vi "Initialize.vi"(7 "Serial Configuration":T1={"Baud Rate"=9600, "Parity"=0, "Data Bits"=8, "Stop Bits"=10, "Flow Control"=0} {"Flow Control" items=["None", "XON/XOFF", "RTS/CTS", "XON/XOFF & RTS/CTS", "DTR/DSR", "XON/XOFF & DTR/DSR"]; "Stop Bits" items=["1.0"=10, "1.5"=15, "2.0"=20]; "Data Bits" items=["7"=7, "8"=8]; "Parity" items=["None", "Odd", "Even", "Mark", "Space"]; "Baud Rate" items=["300"=300, "600"=600, "1200"=1200, "2400"=2400, "4800"=4800, "9600"=9600, "19200"=19200]}, 8 "error in (no error)":errorcluster, 9 "Reset (True)":bool=TRUE, 10 "ID Query (True)":bool=TRUE, 11 "VISA resource name":refnum<visa-resource-name>) -> (0 "error out":errorcluster, 3 "VISA resource name out":refnum<visa-resource-name>)   [LabVIEW 2024, in "Keithley 648X Series.lvlib"]
doc: "Establishes communication with the instrument and optionally performs an instrument identification query and/or an instrument reset. It also places the instrument in a default state needed for other instrument driver operations. Therefore, call this VI before calling other instrument driver VIs for this instrument. Generally, you need to call the <b>Initialize</b> VI only once at the beginning of an application."
uses:
  <instrlib>/Keithley 648X Series/Keithley 648X Series.lvlib
panel:
  # "(c) 2017 National Instruments.  ALL RIGHTS RESERVED."
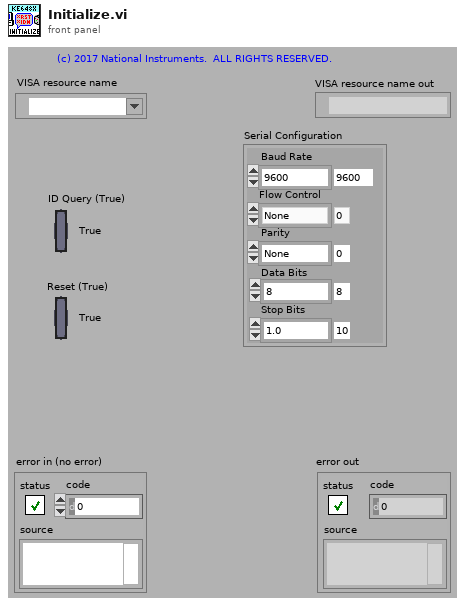
[diagram p1: front panel]
types:
  T1 = cluster{"Baud Rate":u32, "Parity":u16, "Data Bits":u16, "Stop Bits":u16, "Flow Control":u16}
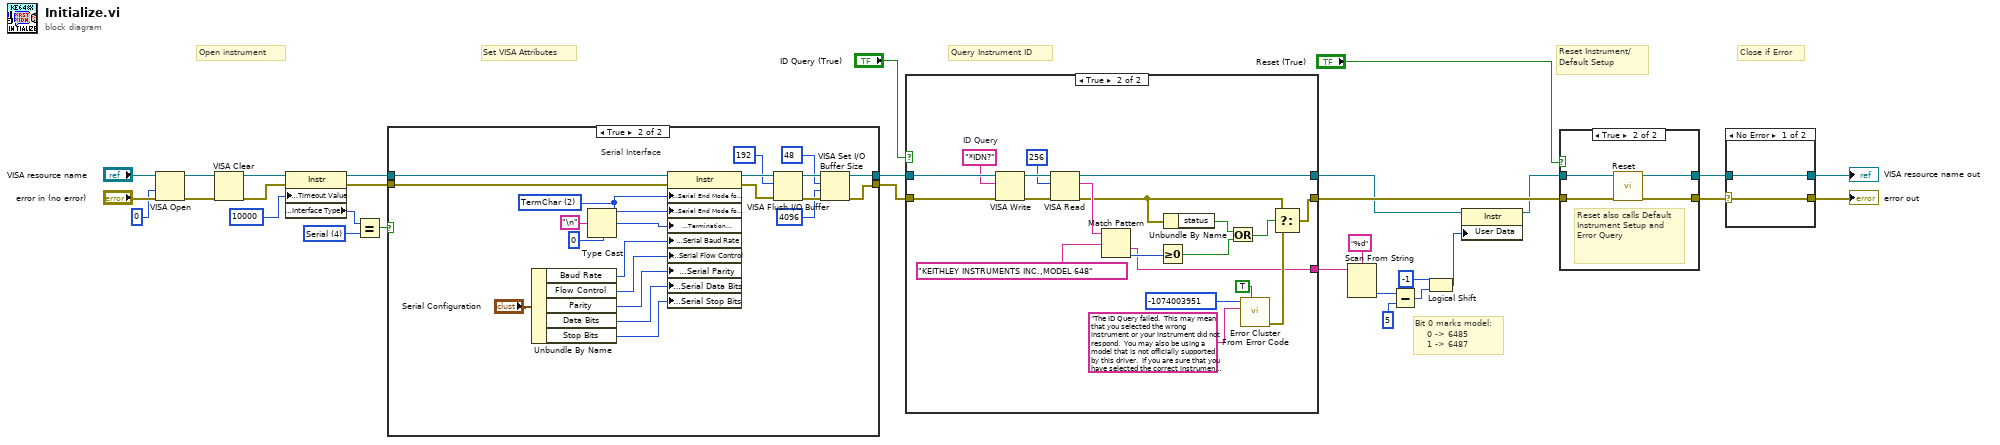
[diagram p0: block diagram]
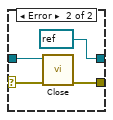
[diagram p3: hidden frame]
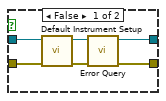
[diagram p4: hidden frame]
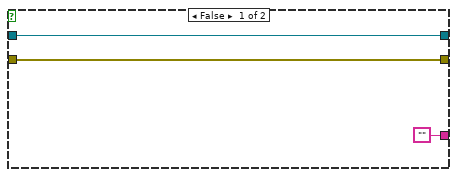
[diagram p5: hidden frame]
diagram:
  w19 = u16 4 items=["GPIB"=1, "VXI"=2, "GPIB-VXI"=3, "Serial"=4, "PXI"=5, "TCPIP"=6, "USB"=7] ("Interface Information:Interface Type")
  # "Bit 0 marks model:\n    0 -> 6485\n    1 -> 6487"
  # "Set VISA Attributes"
  # "Close if Error"
  # "Query Instrument ID"
  # "Reset Instrument/\nDefault Setup"
  # "Open instrument"
  n1 = VISA Open(access mode=u32 0, error in (no error)="error in (no error)", VISA resource name="VISA resource name") -> (VISA resource name=w17:refnum<visa-resource-name>, error out=w16:errorcluster)  [unwired: 2 in]
  n2 = VISA Clear(VISA resource name=w17, error in (no error)=w16) -> (VISA resource name out=w15:refnum<visa-resource-name>, error out=w14:errorcluster)
  n3 = property class="Instr"(reference=w15, error in=w14, "General Settings:Timeout Value"=u32 10000) -> (reference out=w22:refnum<visa-resource-name>, error out=w21:errorcluster, "Interface Information:Interface Type"=w26:u16)
  n4 = Equal?(x=w26, y=w19) -> (x = y?=w20:bool)
  n5 = case shown="True" w20 {
    tunnel: [w32 w51] -> w24
    tunnel: [w33 w48] -> w23
    tunnel: w22 -> [w32 w53]
    tunnel: w21 -> [w33 w54]
    frame False {
      # "GPIB Interface"
    }
    frame True {
      w41 = u16 2 items=["None", "LastBit", "TermChar"] ("Serial Settings:Serial End Mode for Reads")
      # "Serial Interface"
      n6 = Unbundle By Name("Serial Configuration") -> ("Baud Rate"=w39:u32, "Flow Control"=w35:u16, "Parity"=w37:u16, "Data Bits"=w38:u16, "Stop Bits"=w34:u16)
      n7 = Type Cast(type=u8 0, x="\n" ("Line Feed Constant")) -> (*(type *) &x=w40:u8)
      n8 = property class="Instr"(reference=w53, error in=w54, "Serial Settings:Serial End Mode for Reads"=w41, "Serial Settings:Serial End Mode for Writes"=w41, "Message Based Settings:Termination Character"=w40, "Serial Settings:Serial Baud Rate"=w39, "Serial Settings:Serial Flow Control"=w35, "Serial Settings:Serial Parity"=w37, "Serial Settings:Serial Data Bits"=w38, "Serial Settings:Serial Stop Bits"=w34) -> (reference out=w47:refnum<visa-resource-name>, error out=w50:errorcluster)
      n9 = VISA Flush I/O Buffer(VISA resource name=w47, mask (16)=u16 192, error in (no error)=w50) -> (VISA resource name out=w52:refnum<visa-resource-name>, error out=w49:errorcluster)
      n10 = VISA Set I/O Buffer Size(VISA resource name=w52, mask (16)=u16 48, size (4096)=u32 4096 ("size (0)"), error in (no error)=w49) -> (VISA resource name out=w51:refnum<visa-resource-name>, error out=w48:errorcluster)
    }
  }
  n11 = case shown="True" "ID Query (True)" {
    tunnel: [w56 w77] -> w31
    tunnel: [w57 w74] -> w7
    tunnel: w24 -> [w57 w75]
    tunnel: w23 -> [w56 w76]
    tunnel: ["" w58] -> w9
    frame False {
    }
    frame True {
      w68 = "*IDN?"  # ID Query
      n12 = VISA Write(VISA resource name=w75, write buffer=w68, error in (no error)=w76) -> (VISA resource name out=w72:refnum<visa-resource-name>, error out=w71:errorcluster)  [unwired: 1 out]
      n13 = VISA Read(VISA resource name=w72, byte count=u32 256, error in (no error)=w71) -> (VISA resource name out=w74:refnum<visa-resource-name>, read buffer=w73:string, error out=w63:errorcluster)  [unwired: 1 out]
      n14 = Match Pattern(string=w73, regular expression="KEITHLEY INSTRUMENTS INC.,MODEL 648") -> (after substring=w58:string, offset past match=w64:i32)  [unwired: 1 in, 2 out]
      n15 = Greater Or Equal To 0?(x=w64) -> (x >= 0?=w61:bool)
      n16 = Unbundle By Name(w63) -> ("status"=w62:bool)
      n17 = Or(x=w62, y=w61) -> (x .or. y?=w60:bool)
      n18 = call <vilib>:"Error Cluster From Error Code.vi"("show call chain? (False)"=TRUE, "error message (\"\")"="The ID Query failed.  This may mean that you selected the wrong instrument or your instrument did not respond.  You may also be using a model that is not officially supported by this driver.  If you are sure that you have selected the correct instrument and it is responding, try disabling the ID Query." ("Source (VI Name)"), "error code (0)"=-1074003951 ("Code")) -> ("error out"=w67:errorcluster)  [unwired: 6 in]
      n19 = Select(t=w63, s=w60, f=w67) -> (s? t:f=w77:errorcluster)
    }
  }
  n20 = Scan From String(format string="%d", input string=w9) -> (output 1=w6:i32)  [unwired: 3 in, 3 out]
  n21 = Subtract(x=w6, y=5) -> (x-y=w3:i32)
  n22 = Logical Shift(y=i16 -1, x=w3) -> (x << y=w4:i32)
  n23 = property class="Instr"(reference=w7, "User Data"=w4) -> (reference out=w1:refnum<visa-resource-name>)  [unwired: 1 in, 1 out]
  n24 = case shown="True" "Reset (True)" {
    tunnel: w31 -> [w82 w84]
    tunnel: [w79 w87] -> w10
    tunnel: w1 -> [w83 w85]
    tunnel: [w80 w86] -> w11
    frame False {
      n25 = call <instrlib>:"Default Instrument Setup.vi"("error in (no error)"=w82, "VISA resource name"=w83) -> ("error out"=w78:errorcluster, "VISA resource name out"=w81:refnum<visa-resource-name>)  [unwired: 8 in]
      n26 = call <instrlib>:"Error Query.vi"("error in (no error)"=w78, "VISA resource name"=w81) -> ("error out"=w79:errorcluster, "VISA resource name out"=w80:refnum<visa-resource-name>)  [unwired: 6 in, 2 out]
    }
    frame True {
      # "Reset also calls Default Instrument Setup and Error Query"
      n27 = call <instrlib>:"Reset.vi"("VISA resource name"=w85, "error in (no error)"=w84) -> ("VISA resource name out"=w86:refnum<visa-resource-name>, "error out"=w87:errorcluster)  [unwired: 12 in]
    }
  }
  n28 = case shown="No Error" w10 {
    selector: w10 -> [w88 w91]
    tunnel: w11 -> [w89 w92]
    tunnel: [w89 refnum<visa-resource-name> refnum ("VISA resource name out")] -> w13
    tunnel: [w88 w93] -> w12
    frame No Error {
    }
    frame Error {
      n29 = call <instrlib>:"Close.vi"("error in (no error)"=w91, "VISA resource name"=w92) -> ("error out"=w93:errorcluster)  [unwired: 9 in]
    }
  }
  "VISA resource name out" <- w13
  "error out" <- w12
